vi "Stage update boundary.vi"(10 "Stage position 2":T1={"X Position"=-1.4181006249999957, "Y Position"=-10.331925468750049, "Z Position"=5.567119999999971}, 11 "Stage position 1":T1={"X Position"=-1.4181006249999957, "Y Position"=-10.331925468750049, "Z Position"=5.567119999999971}) -> ()   [LabVIEW 2020]
uses:
  typedefs/typedef_boundaries.ctl
  typedefs/typedef_stage_position.ctl
  Global stage boundaries.vi
panel:
  in  "Stage boundary positions":T2={"X lower bound"=-40.0, "X upper bound"=2.6, "Y lower bound"=4.66, "Y upper bound "=12.78, "Z lower bound"=-0.001, "Z upper bound "=8.0}
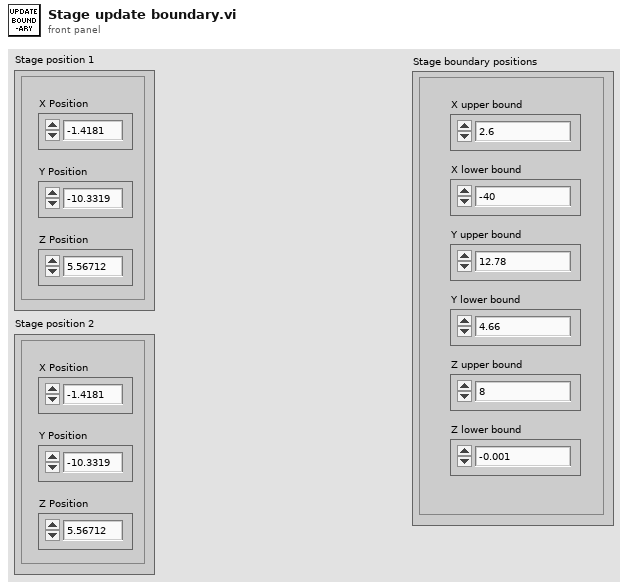
[diagram p1: front panel]
types:
  T1 = typedef "typedef_stage_position.ctl" = cluster{"X Position":dbl, "Y Position":dbl, "Z Position":dbl}
  T2 = typedef "typedef_boundaries.ctl" = cluster{"X lower bound":dbl, "X upper bound":dbl, "Y lower bound":dbl, "Y upper bound ":dbl, "Z lower bound":dbl, "Z upper bound ":dbl}
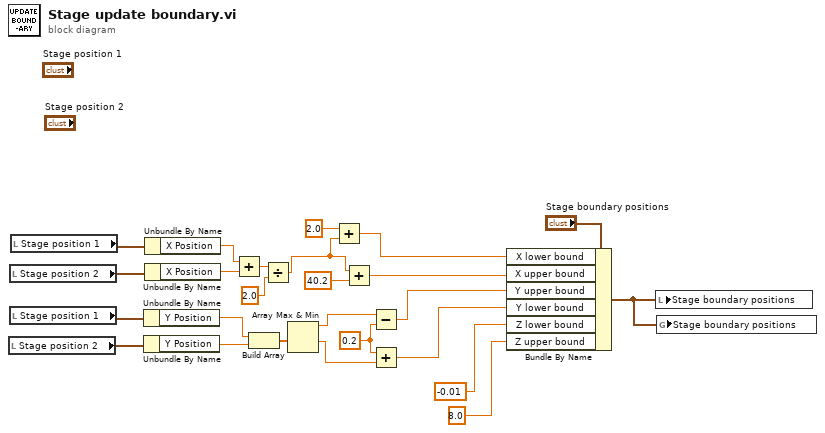
[diagram p0: block diagram]
diagram:
  w5 = 0.2 ("x")
  n1 = local read "Stage position 2"() -> (w17:T1)
  n2 = local read "Stage position 2"() -> (w23:T1)
  n3 = local read "Stage position 1"() -> (w16:T1)
  n4 = local read "Stage position 1"() -> (w24:T1)
  n5 = Unbundle By Name(w16) -> ("Y Position"=w14:dbl)
  n6 = Unbundle By Name(w17) -> ("Y Position"=w13:dbl)
  n7 = Unbundle By Name(w24) -> ("X Position"=w22:dbl)
  n8 = Unbundle By Name(w23) -> ("X Position"=w21:dbl)
  n9 = Add(x=w22, y=w21) -> (x+y=w20:dbl)
  n10 = Build Array(w14, w13) -> (w12:dbl[])
  n11 = Divide(x=w20, y=2.0) -> (x/y=w9:dbl)
  n12 = Array Max & Min(array=w12) -> (max value=w4:dbl, min value=w6:dbl)  [unwired: 2 out]
  n13 = Add(x=2.0, y=w9) -> (x+y=w7:dbl)
  n14 = Add(x=w9, y=40.2) -> (x+y=w19:dbl)
  n15 = Subtract(x=w4, y=w5) -> (x-y=w3:dbl)
  n16 = Add(x=w5, y=w6) -> (x+y=w2:dbl)
  n17 = Bundle By Name(cluster="Stage boundary positions", "X lower bound"=w7, "X upper bound"=w19, "Y upper bound"=w3, "Y lower bound"=w2, "Z lower bound"=-0.01, "Z upper bound"=8.0) -> (w1:T2)
  n18 = local write "Stage boundary positions"(w1) -> ()
  n19 = global write "Global stage boundaries.vi" "Stage boundary positions"(w1) -> ()
